vi "Move XYZOAT.vi"(3 "Make Vertical":bool, 4 "Side":T2=enum."right", 5 "Label":string, 6 "Wait Time":dbl, 8 "error in":errorcluster, 9 "Speed (mm/s)":dbl=50.0, 10 "XYZOAT":T1, 11 "Location":string) -> (0 "error out":errorcluster)   [LabVIEW 2013]
uses:
  ROS/Code/SubVIs/BaxterSide.ctl
  Move Matrix.vi
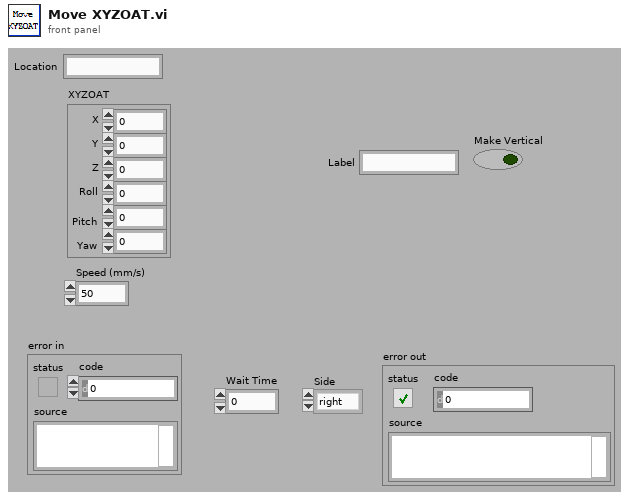
[diagram p1: front panel]
types:
  T1 = cluster{"X":dbl, "Y":dbl, "Z":dbl, "Roll":dbl, "Pitch":dbl, "Yaw":dbl}
  T2 = typedef "BaxterSide.ctl" = enum16{"left", "right"}
  T3 = typedef "NI_Matrix.lvlib/RealMatrix.ctl" = dbl[][]
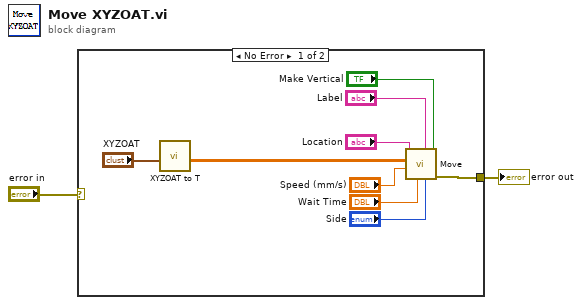
[diagram p0: block diagram]
diagram:
  n1 = case shown="No Error" "error in" {
    selector: "error in" -> [_ w12]
    tunnel: [w10 w12] -> w1
    frame No Error {
      n2 = call "XYZOAT to T.vi"("XYZOAT"="XYZOAT") -> ("T"=w6:T3)  [unwired: 10 in]
      n3 = call-poly "Move.vi"("Make Vertical"="Make Vertical", "Side"="Side", "Label"="Label", "Wait Time"="Wait Time", "Speed (mm/s)"="Speed (mm/s)", "Offset"=w6, "Location"="Location") -> ("error out"=w10:errorcluster)  [unwired: 4 in]
    }
    frame Error {
    }
  }
  "error out" <- w1
